vi "Helper - Check for irons.vi"(9 "Angle to check":dbl, 10 "Wind - Irons range":dbl, 11 "Wind + Irons range":dbl) -> (2 "In irons?":bool)   [LabVIEW 2011]
doc: "Takes in wind angle + irons range and wind angle - irons range, both normalized to be within 0-360, and checks whether the angle inputed falls within the irons range."
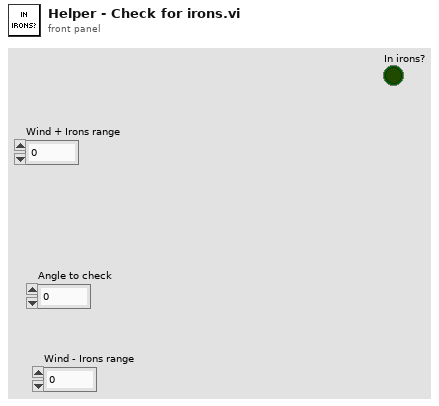
[diagram p1: front panel]
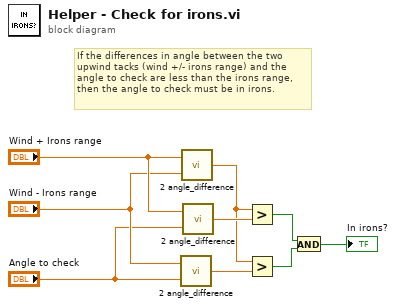
[diagram p0: block diagram]
diagram:
  # "If the differences in angle between the two\nupwind tacks (wind +/- irons range) and the\nangle to check are less than the irons range,\nthen the angle to check must be in irons."
  n1 = call "2 angle_difference.vi"("Angle 2"="Angle to check", "Angle 1"="Wind - Irons range") -> ("Difference"=w5:dbl)
  n2 = call "2 angle_difference.vi"("Angle 2"="Wind - Irons range", "Angle 1"="Wind + Irons range") -> ("Difference"=w4:dbl)
  n3 = call "2 angle_difference.vi"("Angle 2"="Angle to check", "Angle 1"="Wind + Irons range") -> ("Difference"=w6:dbl)
  n4 = Greater?(x=w4, y=w6) -> (0:w2:bool)
  n5 = Greater?(x=w4, y=w5) -> (0:w3:bool)
  n6 = And(x=w2, y=w3) -> (x .and. y?=→"In irons?":bool)
